vi "2D experiment kinect.vi"() -> ()   [LabVIEW 2011]
uses:
  <vilib>/Platform/TimedLoop/XDataNode/timing_clust.ctl
  <vilib>/Platform/TimedLoop/XDataNode/nitl_modes.ctl
  <vilib>/Platform/TimedLoop/XDataNode/wakeup.ctl
  <vilib>/Utility/cursorutil.llb/Set Cursor (Cursor ID).vi
  <vilib>/Utility/inputDevices.llb/closeMouse.vi
  <vilib>/Utility/inputDevices.llb/mouseAcquire.vi
  <vilib>/Utility/file.llb/Write To Spreadsheet File (DBL).vi
  <vilib>/Utility/file.llb/Write To Spreadsheet File (I64).vi
  <vilib>/Platform/TimedLoop/XDataNode/XDataNode.xnode
  User32.dll
  <vilib>/Platform/TimedLoop/XDataNode/XDNodeRunTimeDep.lvlib
  3D_Experiment/kinect-1-4/Kinect_API.lvlib
panel:
  in  "Far object filter 2":i32(slide)=26869 scale=0.0..4305.0
  out "click 2":bool
  in  "Replace with?":i32=60000
  out "stop":bool
  out "initial time":u32
  out "XY Graph":cluster{"Y":dbl[], "Y":dbl[]}[](graph)
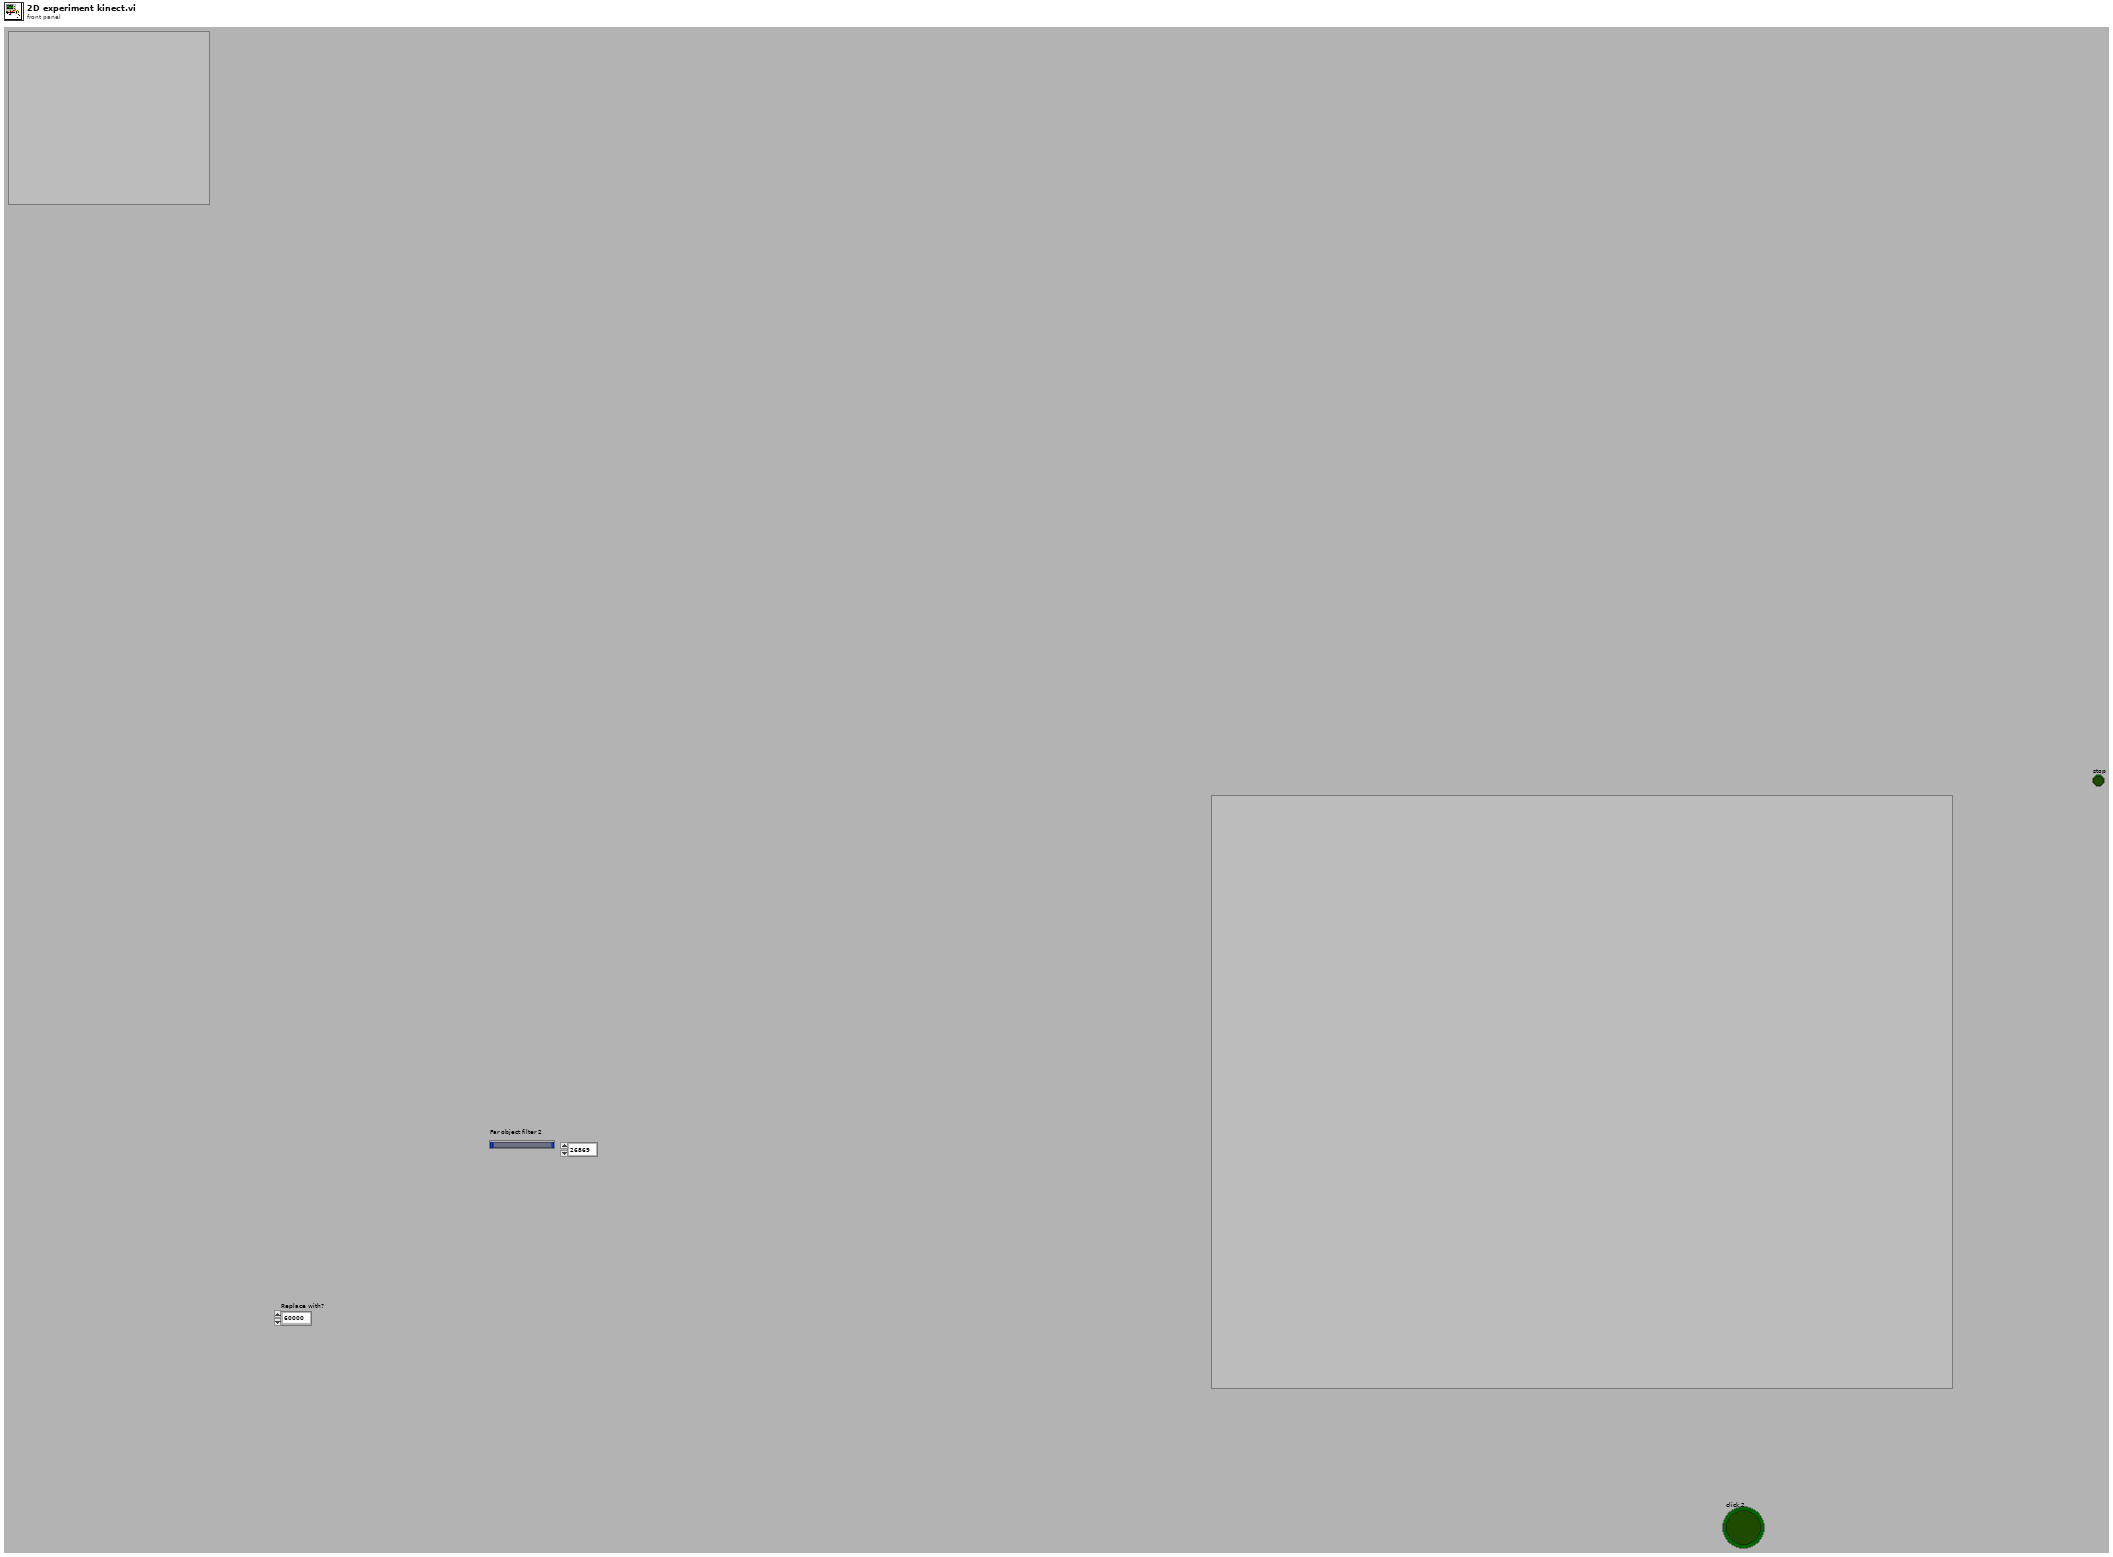
[diagram p1: front panel]
types:
  T1 = enum16{"open", "replace", "create", "open or create", "replace or create", "replace or create with confirmation"}
  T2 = typedef "XDNodeRunTimeDep.lvlib/timing_clust.ctl" = cluster{"Expected End [f-1]":u64, "Actual End [f-1]":u64, "Finished Late? [f-1]":bool, "Expected End [i-1]":u64, "Actual End [i-1]":u64, "Finished Late? [i-1]":bool, "Expected Start [i]":u64, "Actual Start [i]":u64, "Expected Start [f]":u64, "Actual Start [f]":u64, "Source Name":string, "Structure Name":string, "Period":i64, "Deadline":i64, "Offset":i64, "Start":i64, "Priority":i32, "Timeout":i32, "Mode":T3, "Wakeup Reason":T4, "Error":errorcluster, "Source Type":string, "Secondary Source Type":string, "Global End Time":u64, "Global Start Time":u64, "Frame Duration":u64, "Iteration Duration":u64, "Assigned CPU":i32, "I/O Scan Engine Mode":u32}
  T3 = typedef "XDNodeRunTimeDep.lvlib/nitl_modes.ctl" = enum32{"No Change", "Process missed periods, maintain original phase", "Discard missed periods, maintain original phase", "Process missed periods, ignore original phase", "Discard missed periods, ignore original phase"}
  T4 = typedef "XDNodeRunTimeDep.lvlib/wakeup.ctl" = enum32{"Normal", "Aborted", "Asynchronous wakeup", "Timing source error", "Timed loop error", "Timeout"}
  T5 = typedef "LVAllMonitorsDisplayTypeDef.ctl" = cluster{"Bounds":cluster{"Left":i16, "Top":i16, "Right":i16, "Bottom":i16}, "Depth":i16}[]
  T6 = cluster{"Bounds":cluster{"Left":i16, "Top":i16, "Right":i16, "Bottom":i16}, "Depth":i16}
  T7 = cluster{"Left":i16, "Top":i16, "Right":i16, "Bottom":i16}
  T8 = cluster{"queue out":refnum<queue>, "queue out":refnum<queue>}
  T9 = cluster{"new reference":refnum<k24>, "DepthStream":refnum<k24>, "VideoStream":refnum<k24>, "Event Callback":refnum<k27>, "Event Callback":refnum<k27>}
  T10 = cluster{"Horizontal":i32, "Vertical":i32, "Scrolling":i32}
  T11 = cluster{"button 1":bool, "button 2":bool, "button 3":bool, "button 4":bool}
  T12 = cluster{"Radius":dbl, "x0":dbl, "y0":dbl, "D":dbl, bool}
  T13 = typedef "LVPoint32TypeDef.ctl" = cluster{"Horizontal":i32, "Vertical":i32}
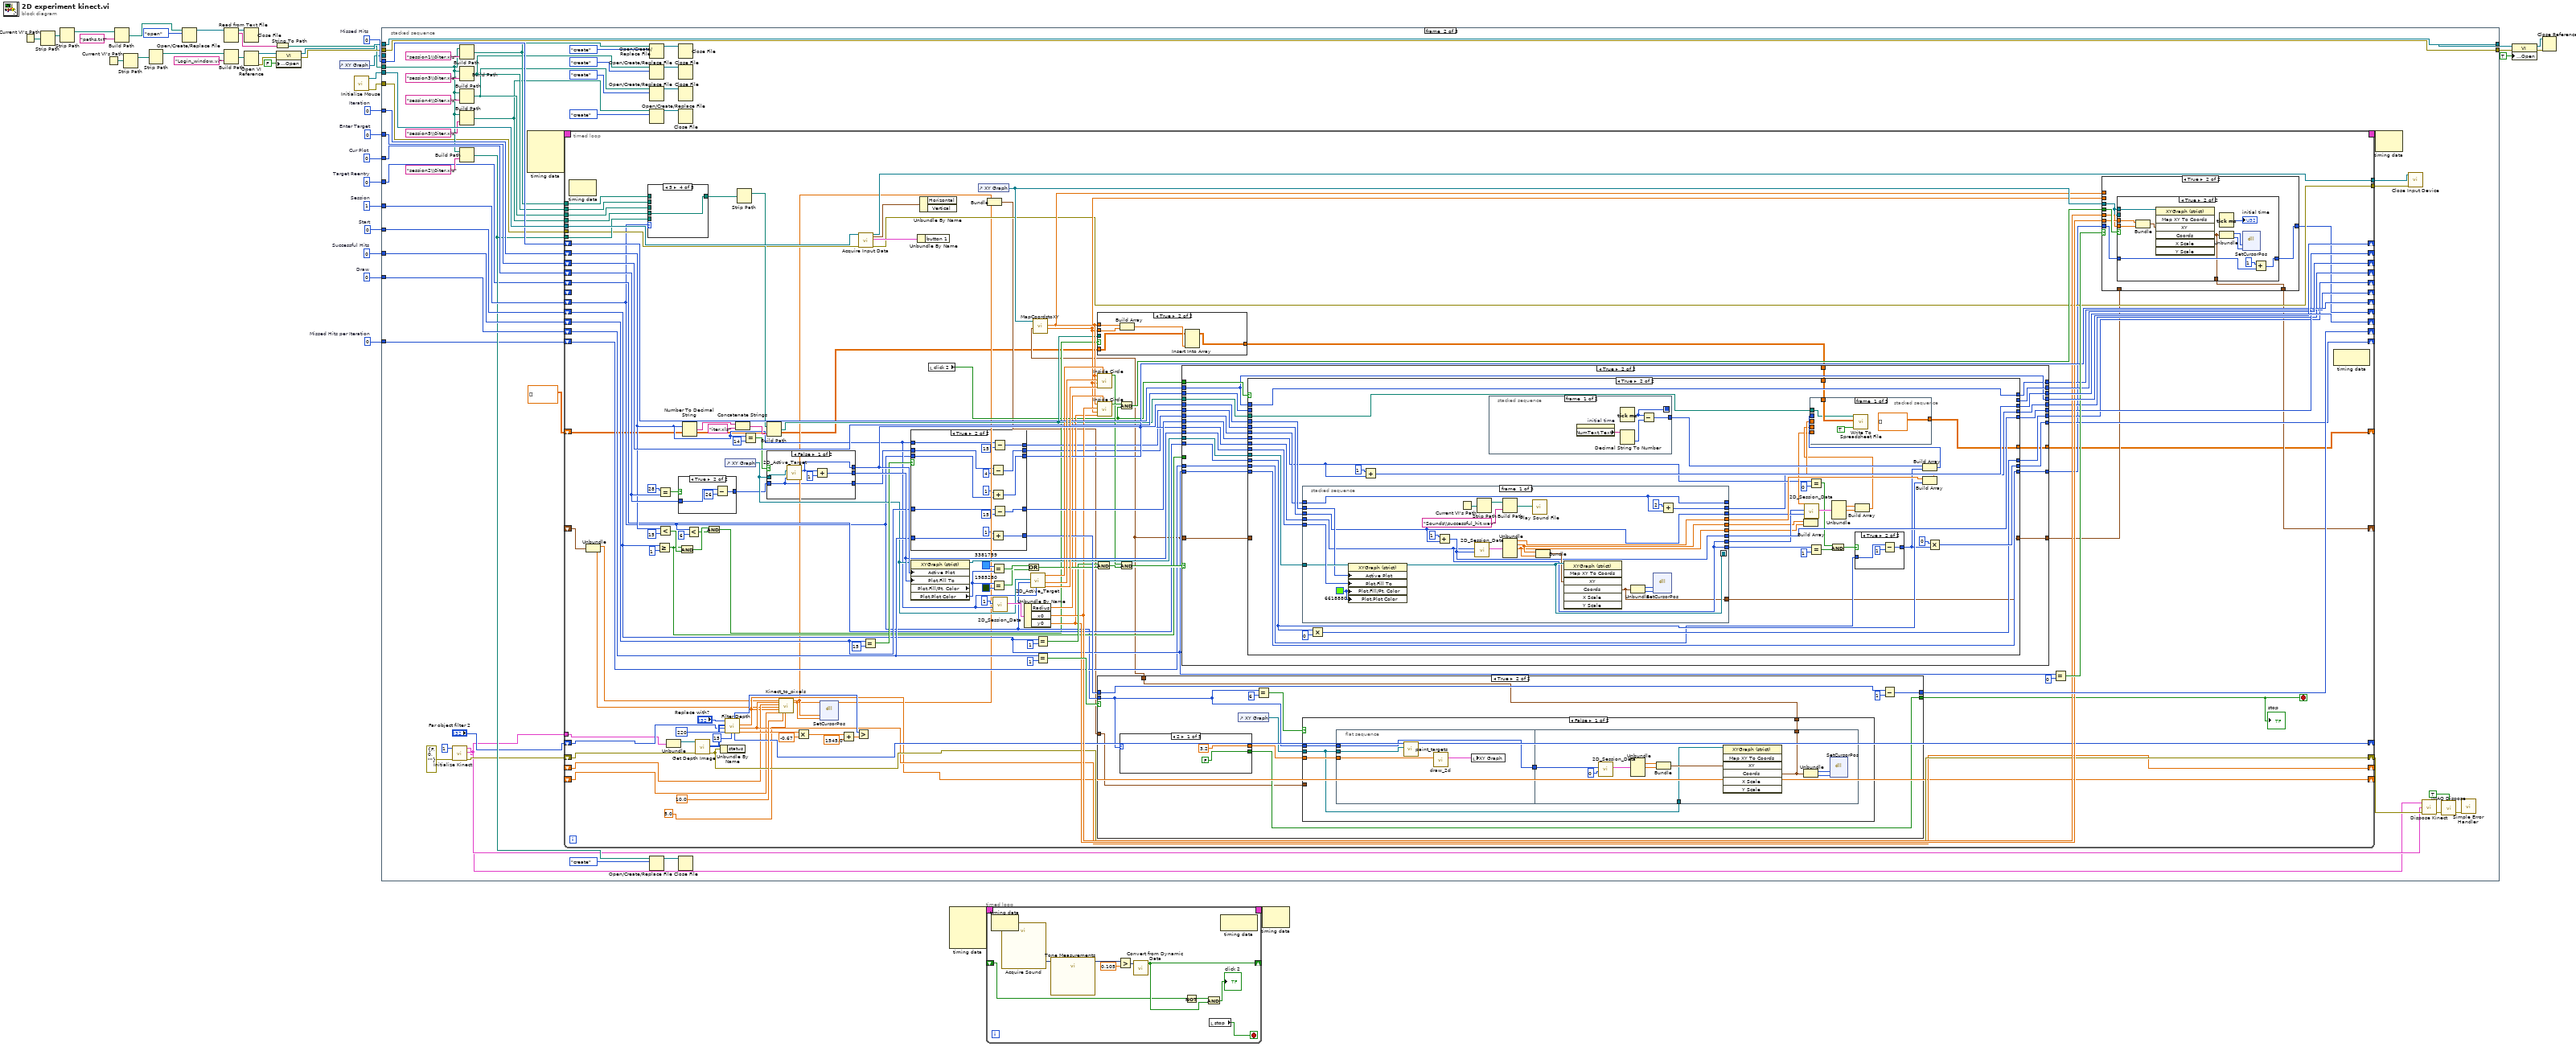
[diagram p0: block diagram]
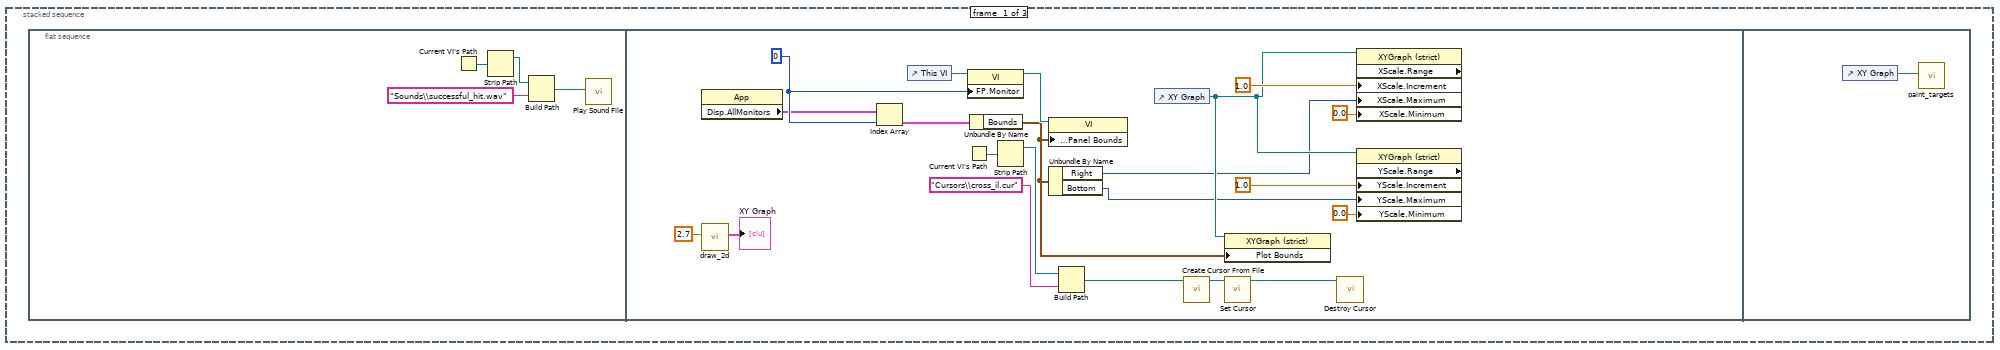
[diagram p2: hidden frame]
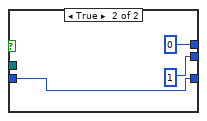
[diagram p8: hidden frame]
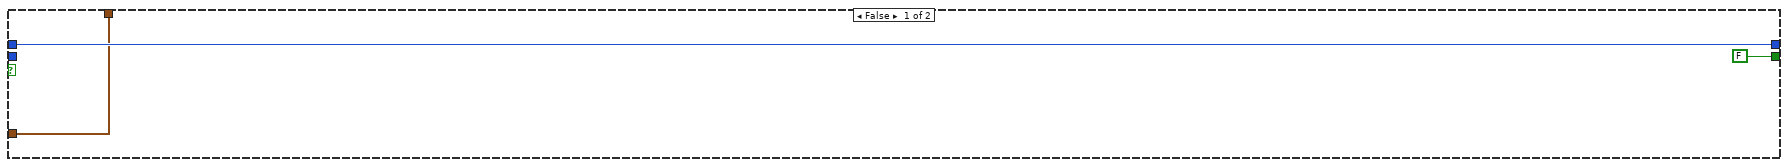
[diagram p10: hidden frame]
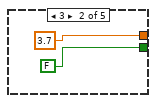
[diagram p12: hidden frame]
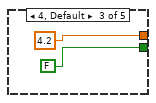
[diagram p13: hidden frame]
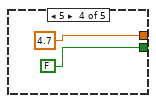
[diagram p14: hidden frame]
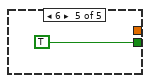
[diagram p15: hidden frame]
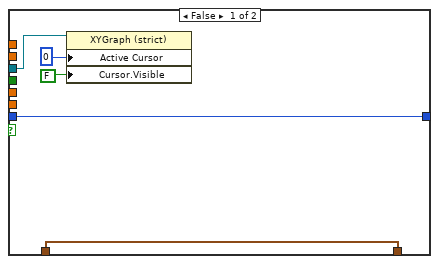
[diagram p16: hidden frame]
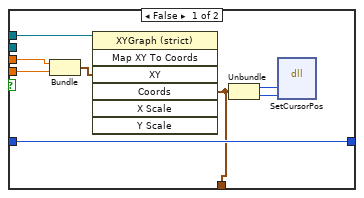
[diagram p17: hidden frame]
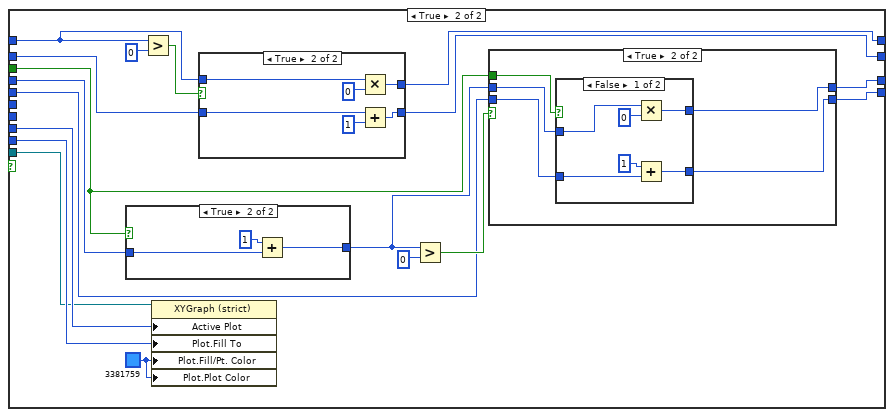
[diagram p20: hidden frame]
diagram:
  w3 = 0  # Target Reentry
  w4 = 0  # Missed Hits per Iteration
  w32 = 0  # Iteration
  w33 = 0  # Cur Plot
  w35 = 0  # Start
  w36 = 0  # Draw
  w37 = 1  # Session
  w38 = 0  # Successful Hits
  w39 = 0  # Missed Hits
  w40 = 0  # Enter Target
  n1 = Current VI's Path() -> (path=w13:path)
  n2 = Strip Path(path=w13) -> (stripped path=w8:path)  [unwired: 1 out]
  n3 = Strip Path(path=w8) -> (stripped path=w7:path)  [unwired: 1 out]
  n4 = Current VI's Path() -> (path=w28:path)
  n5 = Build Path(base path=w7, name or relative path="paths.txt") -> (appended path=w12:path)
  n6 = Strip Path(path=w28) -> (stripped path=w23:path)  [unwired: 1 out]
  n7 = Strip Path(path=w23) -> (stripped path=w22:path)  [unwired: 1 out]
  n8 = Open/Create/Replace File(file path (use dialog)=w12, operation (0:open)=T1."open") -> (refnum out=w15:refnum<file>)  [unwired: 4 in, 2 out]
  n9 = Read from Text File(file (use dialog)=w15) -> (refnum out=w16:refnum<file>, text=w14:string)  [unwired: 3 in, 2 out]
  n10 = Build Path(base path=w22, name or relative path="Login_window.vi") -> (appended path=w26:path)
  n11 = Close File(refnum=w16) -> ()  [unwired: 1 in, 2 out]
  n12 = Open VI Reference(vi path=w26) -> (vi reference=w31:refnum<vi>, error out=w30:errorcluster)  [unwired: 5 in]
  n13 = String To Path(string=w14) -> (path=w9:path)
  n14 = property class="VI"(reference=w31, error in=w30, "Front Panel Window:Open"=FALSE) -> (reference out=w25:refnum<vi>, error out=w24:errorcluster)
  n15 = control-ref of="XY Graph"() -> (w6:refnum<vi>)
  n16 = call <vilib>:"Initialize Mouse.vi"() -> ("error out"=w5:errorcluster, "device ID"=w34:refnum<k1>)  [unwired: 10 in]
  n17 = stacked-sequence {
    tunnel: w34 -> [_ w116 _]
    tunnel: w38 -> [_ w115 _]
    tunnel: w39 -> [_ w114 _]
    tunnel: w37 -> [_ w110 _]
    tunnel: w35 -> [_ w113 _]
    tunnel: w36 -> [_ w112 _]
    tunnel: w40 -> [_ w111 _]
    tunnel: w33 -> [_ w109 _]
    tunnel: w32 -> [_ w108 _]
    tunnel: w25 -> [_ w105 _]
    tunnel: w24 -> [_ w104 _]
    tunnel: [_ w105 _] -> w18
    tunnel: [_ w104 _] -> w17
    tunnel: w9 -> [_ w85 _]
    tunnel: w6 -> [_ _ w588]
    tunnel: w5 -> [_ w78 _]
    tunnel: w4 -> [_ w89 _]
    tunnel: w3 -> [_ w88 _]
    frame #0 {
      n18 = flat-sequence {
        frame #0 {
          n19 = Current VI's Path() -> (path=w42:path)
          n20 = Strip Path(path=w42) -> (stripped path=w43:path)  [unwired: 1 out]
          n21 = Build Path(base path=w43, name or relative path="Sounds\\successful_hit.wav") -> (appended path=w41:path)
          n22 = call <vilib>:"Play Sound File.vi"("path"=w41) -> ()  [unwired: 9 in, 2 out]
        }
        frame #1 {
          w61 = u16 0 ("Front Panel Window:Monitor")
          n23 = property class="App"() -> ("Disp.AllMonitors"=w60:T5)  [unwired: 2 in, 2 out]
          n24 = call "draw_2d.vi"("ID"=2.7) -> ("appended array"=→"XY Graph":cluster{dbl[], dbl[]}[])  [unwired: 10 in]
          n25 = Index Array(array=w60, index=w61) -> (element=w62:T6)
          n26 = control-ref of="This VI"() -> (w63:refnum<vi>)
          n27 = Current VI's Path() -> (path=w52:path)
          n28 = property class="VI"(reference=w63, "FP.Monitor"=w61) -> (reference out=w59:refnum<vi>)  [unwired: 1 in, 1 out]
          n29 = Unbundle By Name(w62) -> ("Bounds"=w58:T7)
          n30 = Strip Path(path=w52) -> (stripped path=w51:path)  [unwired: 1 out]
          n31 = property class="VI"(reference=w59, "Front Panel Window:Panel Bounds"=w58) -> ()  [unwired: 1 in, 2 out]
          n32 = Unbundle By Name(w58) -> ("Right"=w46:i16, "Bottom"=w45:i16)
          n33 = Build Path(base path=w51, name or relative path="Cursors\\cross_il.cur") -> (appended path=w49:path)
          n34 = control-ref of="XY Graph"() -> (w53:refnum<vi>)
          n35 = call <vilib>:"Create Cursor From File.vi"("cursor file"=w49) -> ("cursor ID"=w48:refnum<k1>)  [unwired: 9 in, 1 out]
          n36 = property on="Property Node" class="XYGraph (strict)"(reference=w53, "Plot Bounds"=w58) -> ()  [unwired: 1 in, 2 out]
          n37 = call-poly <vilib>:"Set Cursor.vi"("cursor ID"=w48) -> ("previous cursor ID"=w47:refnum<k1>)  [unwired: 9 in, 1 out]
          n38 = call <vilib>:"Destroy Cursor.vi"("cursor ID"=w47) -> ()  [unwired: 9 in, 1 out]
          n39 = property on="Property Node" class="XYGraph (strict)" props=["XScale", "Range", "XScale", "Increment", "XScale", "Maximum", "XScale", "Minimum"](reference=w53, "XScale.Increment"=1.0 ("X Scale.Range:Increment"), "XScale.Maximum"=w46, "XScale.Minimum"=0.0 ("X Scale.Range:Minimum")) -> ()  [unwired: 1 in, 3 out]
          n40 = property on="Property Node" class="XYGraph (strict)" props=["YScale", "Range", "YScale", "Increment", "YScale", "Maximum", "YScale", "Minimum"](reference=w53, "YScale.Increment"=1.0 ("Y Scale.Range:Increment"), "YScale.Maximum"=w45, "YScale.Minimum"=0.0 ("Y Scale.Range:Minimum")) -> ()  [unwired: 1 in, 3 out]
        }
        frame #2 {
          n41 = control-ref of="XY Graph"() -> (w66:refnum<vi>)
          n42 = call "paint_targets.vi"("XYGraph Refnum"=w66) -> ()  [unwired: 11 in]
        }
      }
    }
    frame #1 {
      n43 = call "Initialize Kinect.vi"("error in (no error)"=errorcluster {"status"=FALSE, "code"=0, "source"=""}, "Buffer Size"=1) -> ("error out"=w71:errorcluster, "Queues Out"=w69:T8, "References"=w68:T9)  [unwired: 7 in]
      n44 = Build Path(base path=w85, name or relative path="session1\\0iter.xls") -> (appended path=w98:path)
      n45 = Build Path(base path=w85, name or relative path="session3\\0iter.xls") -> (appended path=w92:path)
      n46 = Build Path(base path=w85, name or relative path="session4\\0iter.xls") -> (appended path=w82:path)
      n47 = Build Path(base path=w85, name or relative path="session5\\0iter.xls") -> (appended path=w79:path)
      n48 = Build Path(base path=w85, name or relative path="session2\\0iter.xls") -> (appended path=w95:path)
      n49 = node-c288() -> (w107:T2)  [unwired: 4 in]
      n50 = timed-loop {
        tunnel: w116 -> [w233]
        tunnel: [w232] -> w91
        shift-right: [w231] -> _
        shift-left: w115 -> [w218]
        shift-right: [w229] -> _
        shift-left: w114 -> [w230]
        shift-right: [w210] -> _
        shift-left: w110 -> [w158]
        shift-right: [w160] -> _
        shift-left: w113 -> [w179]
        shift-right: [w215] -> _
        shift-left: w112 -> [w216]
        shift-right: [w211] -> _
        shift-left: w111 -> [w212]
        shift-right: [w196] -> _
        shift-left: w108 -> [w170]
        shift-right: [w195] -> _
        shift-left: w109 -> [w192]
        timing: w107 -> [_]
        timing-out: [_] -> w106
        tunnel: w98 -> [w185]
        tunnel: w95 -> [w184]
        tunnel: w92 -> [w183]
        shift-right: [w172] -> _
        shift-left: _ -> [_]
        tunnel: w78 -> [w168]
        tunnel: [w167] -> w90
        shift-right: [w165] -> _
        shift-left: w89 -> [w166]
        shift-right: [w162] -> _
        shift-left: w88 -> [w164]
        tunnel: w82 -> [w154]
        tunnel: w79 -> [w153]
        shift-right: [w138] -> w72
        shift-left: w71 -> [w137]
        shift-right: [w136] -> _
        shift-left: "Far object filter 2" -> [w135]
        tunnel: w69 -> [w134]
        shift-right: [w133] -> _
        shift-left: _ -> [w132]
        shift-right: [w131] -> _
        shift-left: _ -> [w130]
        shift-right: [w124] -> _
        shift-left: _ -> [w123]
        shift-right: [w117] -> _
        shift-left: dbl[][] [] -> [w119]
        stop <- w152 stop-if-true
        n51 = node-c288() -> ()  [unwired: 1 in, 1 out]
        n52 = Unbundle(w123) -> ("X_pixels"=w122:dbl, "Y_pixels"=w121:dbl)
        n53 = case shown="5" w158 {
          tunnel: w185 -> [_ _ _ _ w254]
          tunnel: [w250 w251 w252 w253 w254] -> w178
          tunnel: w184 -> [w250 _ _ _ _]
          tunnel: w183 -> [_ w251 _ _ _]
          tunnel: w154 -> [_ _ w252 _ _]
          tunnel: w153 -> [_ _ _ w253 _]
          frame 2 {
          }
          frame 3 {
          }
          frame 4 {
          }
          frame 5 {
          }
          frame 1, Default {
          }
        }
        n54 = Greater Or Equal?(x=w179, y=1) -> (x >= y?=w163:bool)
        n55 = Equal?(x=28, y=w192) -> (x = y?=w193:bool)
        n56 = Less?(x=w170, y=15) -> (x < y?=w169:bool)
        n57 = Unbundle(w134) -> ("queue out"=w139:refnum<queue>)  [unwired: 1 out]
        n58 = case shown="True" w193 {
          tunnel: w192 -> [w265 w268]
          tunnel: [w265 w266] -> w191
          frame False {
          }
          frame True {
            n59 = Subtract(x=w268, y=26) -> (x-y=w266:i32)
          }
        }
        n60 = And(x=w163, y=w169) -> (x .and. y?=w159:bool)
        n61 = Number To Decimal String(number=w170) -> (decimal integer string=w174:string)  [unwired: 1 in]
        n62 = Less?(x=w158, y=6) -> (x < y?=w156:bool)
        n63 = call "Get Depth Image.vi"("error in (no error)"=w137, "queue in"=w139) -> ("error out"=w138:errorcluster, "Depth Image Pixels (U16)"=w141:u16[][])  [unwired: 6 in, 2 out]
        n64 = And(x=w159, y=w156) -> (x .and. y?=w155:bool)
        n65 = Unbundle By Name(w138) -> ()  [unwired: 1 out]
        n66 = control-ref of="XY Graph"() -> (w199:refnum<vi>)
        n67 = call "Filter Depth.vi"("Wall-Threshold"=15, "Y-Threshold"=220, "Far object filter"=w135, "Depth Image Pixels (U16)"=w141, "Replace with?"="Replace with?") -> ("average Z"=w147:dbl, "average Y"=w133:dbl, "average X"=w131:dbl, "New far object filter"=w136:i32, "Area"=w148:i32)  [unwired: 1 in, 1 out]
        n68 = Concatenate Strings(w174, "iter.xls" ("name or relative path")) -> (w176:string)
        n69 = Strip Path(path=w178) -> (stripped path=w175:path)  [unwired: 1 out]
        n70 = Equal?(x=w170, y=14) -> (x = y?=w189:bool)
        n71 = Build Path(base path=w175, name or relative path=w176) -> (appended path=w173:path)
        n72 = case shown="False" w189 {
          tunnel: [w260 u32 0 ("Active Plot")] -> w238
          tunnel: [w259 u32 1] -> w237
          tunnel: w199 -> [w258 _]
          tunnel: w191 -> [w257 w262]
          tunnel: [w257 w262] -> w188
          frame False {
            n73 = call "2D_Active_Target.vi"("Active Plot"=w257, "XYGraph Refnum"=w258) -> ("Active Plot"=w260:u32)  [unwired: 6 in, 3 out]
            n74 = Add(x=w260, y=u32 1) -> (x+y=w259:u32)
          }
          frame True {
          }
        }
        n75 = call "Kinect_to_pixels.vi"("previous_X_pixels"=w122, "current_X_kinect"=w133, "previous_X_kinect"=w132, "previous_Y_pixels"=w121, "current_Y_kinect"=w131, "previous_Y_kinect"=w130, "X_Y_speed"=10.0, "min_diff"=5.0) -> ("X_pixels"=w129:dbl, "Y_pixels"=w128:dbl)  [unwired: 8 in, 2 out]
        n76 = Multiply(x=w147, y=-0.67 ("x")) -> (x*y=w143:dbl)
        n77 = dll-call lib="User32.dll" fn="SetCursorPos"(w129, w128) -> ()  [unwired: 6 in, 2 out]
        n78 = Add(x=w143, y=1545.0 ("x")) -> (x+y=w144:dbl)
        n79 = Greater?(x=w148, y=w144) -> ()  [unwired: 1 out]
        n80 = call-poly <vilib>:"Acquire Input Data.vi"("device ID"=w233, "error in (no error)"=w168) -> ("device ID"=w232:refnum<k1>, "axis info"=w198:T10, "button info"=w234:T11, "error out"=w167:errorcluster)  [unwired: 1 in, 13 out]
        n81 = Equal?(x=w218, y=15) -> (x = y?=w227:bool)
        n82 = case shown="True" w227 {
          tunnel: w218 -> [w347 w362]
          tunnel: [w347 w361] -> w226
          tunnel: w158 -> [w346 w360]
          tunnel: [w346 w358] -> w210
          tunnel: w216 -> [w345 w357]
          tunnel: [w345 w355] -> w214
          tunnel: w188 -> [w344 w354]
          tunnel: [w344 w352] -> w187
          tunnel: w170 -> [w343 w351]
          tunnel: [w343 w349] -> w186
          frame False {
          }
          frame True {
            n83 = Subtract(x=w354, y=4) -> (x-y=w352:i32)
            n84 = Add(x=1, y=w360) -> (x+y=w358:i32)
            n85 = Add(x=1, y=w357) -> (x+y=w355:i32)
            n86 = Subtract(x=w351, y=15) -> (x-y=w349:i32)
            n87 = Subtract(x=w362, y=15) -> (x-y=w361:i32)
          }
        }
        n88 = property on="Property Node" class="XYGraph (strict)" props=["Active Plot", "Plot", "Fill To", "Plot", "Fill/Pt. Color", "Plot", "Plot Color"](reference=w199, "Active Plot"=w238, "Plot.Fill To"=w237) -> (reference out=w219:refnum<vi>, "Plot.Plot Color"=w220:u32)  [unwired: 1 in, 2 out]
        n89 = Unbundle By Name(w234) -> ()  [unwired: 1 out]
        n90 = Unbundle By Name(w198) -> ()  [unwired: 2 out]
        n91 = local read "click 2"() -> (w151:bool)
        n92 = control-ref of="XY Graph"() -> (w197:refnum<vi>)
        n93 = Bundle("X_pixels"=w129, "Y_pixels"=w128) -> (w127:cluster{"X_pixels":dbl, "Y_pixels":dbl})  [unwired: 1 in]
        n94 = Equal?(x=u32 3381759, y=w220) -> (x = y?=w240:bool)
        n95 = Equal?(x=w220, y=u32 1985280) -> (x = y?=w239:bool)
        n96 = call "2D_Session_Data.vi"("Iteration"=w170, "Session"=1) -> ("output cluster"=w204:T12)  [unwired: 9 in]
        n97 = Unbundle By Name(w204) -> ("Radius"=w203:dbl, "x0"=w202:dbl, "y0"=w201:dbl)
        n98 = Or(x=w240, y=w239) -> (x .or. y?=w208:bool)
        n99 = call "2D_Active_Target.vi"("Iteration"=w170, "Session"=w158, "XYGraph Refnum"=w199) -> ("y0"=w235:dbl, "x0"=w236:dbl, "Radius"=w225:dbl)  [unwired: 5 in, 1 out]
        n100 = Equal?(x=w179, y=1) -> (x = y?=w206:bool)
        n101 = Equal?(x=w216, y=1) -> (x = y?=w213:bool)
        n102 = And(x=w206, y=w208) -> (x .and. y?=w205:bool)
        n103 = case shown="True" w213 {
          tunnel: w158 -> [_ w274]
          tunnel: [w270 w281] -> w215
          tunnel: w214 -> [w270 w280]
          tunnel: [FALSE ("Valid") w278] -> w152
          tunnel: w127 -> [w269 w272]
          tunnel: [w269 w273] -> w126
          frame False {
          }
          frame True {
            n104 = case shown="2" w274 {
              tunnel: [3.2 ("ID") 3.7 ("ID") 4.2 ("ID") 4.7 ("ID") _] -> w279
              tunnel: [FALSE FALSE FALSE FALSE TRUE] -> w278
              frame 2 {
              }
              frame 3 {
              }
              frame 4, Default {
              }
              frame 5 {
              }
              frame 6 {
              }
            }
            n105 = control-ref of="XY Graph"() -> (w275:refnum<vi>)
            n106 = Equal?(x=w274, y=6) -> (x = y?=w276:bool)
            n107 = case shown="False" w276 {
              tunnel: w279 -> [w287 _]
              tunnel: w275 -> [w284 _]
              tunnel: w274 -> [w285 _]
              tunnel: [w283 w302] -> w273
              tunnel: w272 -> [_ w302]
              frame False {
                n108 = flat-sequence {
                  tunnel: w287 -> [w290]
                  tunnel: w284 -> [w289]
                  tunnel: [w288] -> w286
                  tunnel: w285 -> [w288]
                  tunnel: w286 -> [w295]
                  tunnel: w284 -> [w293]
                  tunnel: [w292] -> w283
                  frame #0 {
                    n109 = call "paint_targets.vi"("XYGraph Refnum"=w289) -> ()  [unwired: 11 in]
                    n110 = call "draw_2d.vi"("ID"=w290) -> ("appended array"=w291:cluster{dbl[], dbl[]}[])  [unwired: 10 in]
                    n111 = local write "XY Graph"(w291) -> ()
                  }
                  frame #1 {
                    n112 = call "2D_Session_Data.vi"("Iteration"=0, "Session"=w295) -> ("output cluster"=w299:T12)  [unwired: 9 in]
                    n113 = Unbundle(w299) -> ("x0"=w298:dbl, "y0"=w296:dbl)  [unwired: 3 out]
                    n114 = Bundle("x0"=w298, "y0"=w296) -> (w297:cluster{"x0":dbl, "y0":dbl})  [unwired: 1 in]
                    n115 = invoke on="Invoke Node" class="XYGraph (strict)" method="Map XY To Coords"(reference=w293, "XY"=w297) -> ("Coords"=w292:T13)  [unwired: 5 in, 6 out]
                    n116 = Unbundle(w292) -> ("Horizontal"=w301:i32, "Vertical"=w300:i32)
                    n117 = dll-call lib="User32.dll" fn="SetCursorPos"(w301, w300) -> ()  [unwired: 6 in, 2 out]
                  }
                }
              }
              frame True {
              }
            }
            n118 = Subtract(x=w280, y=1) -> (x-y=w281:i32)
          }
        }
        "stop" <- w152
        n119 = call "MapCoordstoXY.vi"("Coordinates"=w126, "XYGraph Refnum"=w197) -> ("Y(graph)"=w181:dbl, "X (graph)"=w182:dbl)  [unwired: 7 in]
        n120 = case shown="True" w155 {
          tunnel: w182 -> [_ w249]
          tunnel: w181 -> [_ w248]
          tunnel: w173 -> [_ _]
          tunnel: w119 -> [w244 w246]
          tunnel: [w244 w245] -> w118
          frame False {
          }
          frame True {
            n121 = Build Array(w249, w248) -> (w247:dbl[])
            n122 = Insert Into Array(array=w246, new element=w247) -> (w245:dbl[][])  [unwired: 2 in]
          }
        }
        n123 = call "Inside Circle.vi"("Radius"=w225, "y0"=w235, "y"=w181, "x0"=w236, "x"=w182) -> ("Inside Circle"=w207:bool)  [unwired: 6 in]
        n124 = call "Inside Circle.vi"("Radius"=w203, "y0"=w201, "y"=w181, "x0"=w202, "x"=w182) -> ("Inside Circle"=w222:bool)  [unwired: 6 in]
        n125 = And(x=w222, y=w151) -> (x .and. y?=w221:bool)
        n126 = And(x=w207, y=w205) -> (x .and. y?=w242:bool)
        n127 = case shown="True" w242 {
          tunnel: w151 -> [w373 w456]
          tunnel: w238 -> [w381 w453]
          tunnel: w237 -> [w380 w452]
          tunnel: w226 -> [w365 w455]
          tunnel: [w365 w454] -> w231
          tunnel: w230 -> [w375 w440]
          tunnel: [w371 w440] -> w229
          tunnel: w179 -> [w379 w451]
          tunnel: [w379 w450] -> w161
          tunnel: w219 -> [w378 w449]
          tunnel: w212 -> [w370 w448]
          tunnel: [_ w447] -> w211
          tunnel: w210 -> [w366 w446]
          tunnel: w186 -> [w377 w445]
          tunnel: [w377 w444] -> w196
          tunnel: w187 -> [w376 w443]
          tunnel: [w376 w442] -> w195
          tunnel: w173 -> [_ w441]
          tunnel: [w375 w439] -> w172
          tunnel: w166 -> [w374 w438]
          tunnel: [w372 w437] -> w165
          tunnel: w164 -> [w368 w436]
          tunnel: w163 -> [w369 _]
          tunnel: [w367 w435] -> w162
          tunnel: w126 -> [w364 w434]
          tunnel: [w364 w433] -> w125
          tunnel: w118 -> [w363 w432]
          tunnel: [w363 w431] -> w117
          frame False {
            n128 = case shown="False" w369 {
              tunnel: w381 -> [_ w402]
              tunnel: w380 -> [_ w401]
              tunnel: w378 -> [_ w400]
              tunnel: w375 -> [w385 w399]
              tunnel: w374 -> [w384 w395]
              tunnel: w373 -> [_ w386]
              tunnel: [w384 w394] -> w372
              tunnel: [w385 w393] -> w371
              tunnel: w370 -> [w382 w390]
              tunnel: w368 -> [w383 w389]
              tunnel: [w383 w388] -> w367
              tunnel: [w382 w387] -> _
              tunnel: w366 -> [_ _]
              tunnel: w365 -> [_ _]
              frame False {
              }
              frame True {
                w403 = u32 3381759
                n129 = case shown="True" w386 {
                  tunnel: w399 -> [w427 w430]
                  tunnel: [w427 w428] -> w396
                  frame False {
                  }
                  frame True {
                    n130 = Add(x=1, y=w430) -> (x+y=w428:i32)
                  }
                }
                n131 = Greater?(x=w390, y=0) -> (0:w391:bool)
                n132 = property on="Property Node" class="XYGraph (strict)"(reference=w400, "Active Plot"=w402, "Plot.Fill To"=w401, "Plot.Fill/Pt. Color"=w403, "Plot.Plot Color"=w403) -> ()  [unwired: 1 in, 2 out]
                n133 = case shown="True" w391 {
                  tunnel: w390 -> [w404 w411]
                  tunnel: w389 -> [w405 w408]
                  tunnel: [w405 w407] -> w388
                  tunnel: [w404 w406] -> w387
                  frame False {
                  }
                  frame True {
                    n134 = Multiply(x=w411, y=0) -> (x*y=w406:i32)
                    n135 = Add(x=w408, y=1) -> (x+y=w407:i32)
                  }
                }
                n136 = Greater?(x=w396, y=0) -> (0:w397:bool)
                n137 = case shown="True" w397 {
                  tunnel: [w412 w418] -> w394
                  tunnel: [w413 w417] -> w393
                  tunnel: w396 -> [w413 w416]
                  tunnel: w395 -> [w412 w415]
                  tunnel: w386 -> [_ w414]
                  frame False {
                  }
                  frame True {
                    n138 = case shown="False" w414 {
                      tunnel: [w423 w425] -> w418
                      tunnel: [w421 w426] -> w417
                      tunnel: w416 -> [w420 w426]
                      tunnel: w415 -> [w419 w425]
                      frame False {
                        n139 = Multiply(x=w420, y=0) -> (x*y=w421:i32)
                        n140 = Add(x=1, y=w419) -> (x+y=w423:i32)
                      }
                      frame True {
                      }
                    }
                  }
                }
              }
            }
          }
          frame True {
            n141 = case shown="True" w456 {
              tunnel: w455 -> [w471 w485]
              tunnel: [w471 w510] -> w454
              tunnel: w453 -> [w470 w514]
              tunnel: w452 -> [w469 w513]
              tunnel: w451 -> [w468 w512]
              tunnel: [w468 w512] -> w450
              tunnel: w449 -> [w467 w511]
              tunnel: w448 -> [w466 _]
              tunnel: [w464 _] -> w447
              tunnel: w446 -> [_ w509]
              tunnel: w445 -> [w463 w508]
              tunnel: [w463 w507] -> w444
              tunnel: w443 -> [w462 w506]
              tunnel: [w462 w476] -> w442
              tunnel: w441 -> [_ w503]
              tunnel: w440 -> [w461 w502]
              tunnel: [w461 w502] -> w439
              tunnel: w438 -> [w460 w478]
              tunnel: [w460 w501] -> w437
              tunnel: w436 -> [w459 w498]
              tunnel: [w459 w496] -> w435
              tunnel: w434 -> [w458 _]
              tunnel: [w458 w475] -> w433
              tunnel: w432 -> [w457 w474]
              tunnel: [w457 w473] -> w431
              frame False {
                w472 = u32 1985280
                n142 = property on="Property Node" class="XYGraph (strict)"(reference=w467, "Active Plot"=w470, "Plot.Fill To"=w469, "Plot.Fill/Pt. Color"=w472, "Plot.Plot Color"=w472) -> ()  [unwired: 1 in, 2 out]
                n143 = Add(x=w466, y=1) -> (x+y=w464:i32)
              }
              frame True {
                n144 = stacked-sequence {
                  seq-local: [w562 _ _] -> [_ w571 w582]
                  tunnel: w514 -> [w561 w570 w584]
                  tunnel: w513 -> [w564 _ w583]
                  tunnel: w511 -> [w563 _ _]
                  tunnel: w509 -> [w543 _ _]
                  tunnel: w508 -> [w546 w569 _]
                  tunnel: [w548 _ _] -> w507
                  tunnel: [w555 _ _] -> _
                  tunnel: w506 -> [w555 _ _]
                  tunnel: [w553 _ _] -> w476
                  tunnel: [w547 _ _] -> w499
                  tunnel: [w546 _ _] -> w494
                  tunnel: [w543 _ _] -> w493
                  tunnel: [w545 _ _] -> w489
                  tunnel: [w544 _ _] -> w488
                  tunnel: [w543 _ _] -> w483
                  tunnel: [w542 _ _] -> w475
                  frame #0 {
                    w565 = u32 6618880
                    n145 = property on="Property Node" class="XYGraph (strict)"(reference=w563, "Active Plot"=w561, "Plot.Fill To"=w564, "Plot.Fill/Pt. Color"=w565, "Plot.Plot Color"=w565) -> (reference out=w562:refnum<vi>)  [unwired: 1 in, 1 out]
                    n146 = Add(x=1, y=w546) -> (x+y=w548:i32)
                    n147 = Current VI's Path() -> (path=w558:path)
                    n148 = call "2D_Session_Data.vi"("Iteration"=w548, "Session"=w543) -> ("output cluster"=w550:T12)  [unwired: 9 in]
                    n149 = Strip Path(path=w558) -> (stripped path=w557:path)  [unwired: 1 out]
                    n150 = Build Path(base path=w557, name or relative path="Sounds\\successful_hit.wav") -> (appended path=w559:path)
                    n151 = Unbundle(w550) -> ("Radius"=w547:dbl, "x0"=w545:dbl, "y0"=w544:dbl)  [unwired: 2 out]
                    n152 = call <vilib>:"Play Sound File.vi"("path"=w559) -> ()  [unwired: 9 in, 2 out]
                    n153 = Bundle("x0"=w545, "y0"=w544) -> (w549:cluster{"x0":dbl, "y0":dbl})  [unwired: 1 in]
                    n154 = invoke on="Invoke Node" class="XYGraph (strict)" method="Map XY To Coords"(reference=w562, "XY"=w549) -> ("Coords"=w542:T13)  [unwired: 5 in, 6 out]
                    n155 = Unbundle(w542) -> ("Horizontal"=w552:i32, "Vertical"=w551:i32)
                    n156 = dll-call lib="User32.dll" fn="SetCursorPos"(w552, w551) -> ()  [unwired: 6 in, 2 out]
                    n157 = Add(x=2, y=w555) -> (x+y=w553:i32)
                  }
                  frame #1 {
                    w573 = u32 3381759
                    n158 = Equal?(x=15, y=w569) -> (x = y?=w567:bool)
                    n159 = case shown="True" w567 {
                      tunnel: [w575 w579] -> w572
                      tunnel: w570 -> [w574 w581]
                      tunnel: [w574 w577] -> w566
                      frame False {
                        n160 = Add(x=w574, y=u32 1) -> (x+y=w575:u32)
                      }
                      frame True {
                        n161 = Subtract(x=w581, y=u32 2) -> (x-y=w577:u32)
                        n162 = Add(x=w577, y=1 ("x")) -> (x+y=w579:u32)
                      }
                    }
                    n163 = property on="Property Node" class="XYGraph (strict)"(reference=w571, "Active Plot"=w566, "Plot.Fill To"=w572, "Plot.Fill/Pt. Color"=w573, "Plot.Plot Color"=w573) -> ()  [unwired: 1 in, 2 out]
                  }
                  frame #2 {
                    w585 = u32 3223857
                    n164 = property on="Property Node" class="XYGraph (strict)"(reference=w582, "Active Plot"=w584, "Plot.Fill To"=w583, "Plot.Fill/Pt. Color"=w585, "Plot.Plot Color"=w585) -> ()  [unwired: 1 in, 2 out]
                  }
                }
                n165 = Multiply(x=w498, y=0) -> (x*y=w496:i32)
                n166 = Add(x=1, y=w485) -> (x+y=w510:i32)
                n167 = stacked-sequence {
                  seq-local: [w536 _] -> [_ w540]
                  tunnel: [w537 _] -> w504
                  frame #0 {
                    n168 = property on="initial time" class="DigNum (strict)"() -> ("NumText.Text"=w539:string)  [unwired: 2 in, 2 out]
                    n169 = Tick Count (ms)() -> (millisecond timer value=w536:u32)
                    n170 = Decimal String To Number(string=w539) -> (number=w538:i32)  [unwired: 2 in, 1 out]
                    n171 = Subtract(x=w536, y=w538) -> (x-y=w537:u32)
                  }
                  frame #1 {
                    n172 = Number To Decimal String(number=w540) -> (decimal integer string=w541:string)  [unwired: 1 in]
                    n173 = property on="initial time" class="DigNum (strict)"("NumText.Text"=w541) -> ()  [unwired: 2 in, 2 out]
                  }
                }
                n174 = Build Array(w489, w488) -> (w486:dbl[])
                n175 = call "2D_Session_Data.vi"("Iteration"=w494, "Session"=w493) -> ("output cluster"=w492:T12)  [unwired: 9 in]
                n176 = Equal?(x=w485, y=0) -> (x = y?=w481:bool)
                n177 = Equal?(x=w483, y=1) -> (x = y?=w480:bool)
                n178 = And(x=w481, y=w480) -> (x .and. y?=w479:bool)
                n179 = Unbundle(w492) -> ("x0"=w491:dbl, "y0"=w490:dbl)  [unwired: 3 out]
                n180 = Build Array(w491, w490) -> (w487:dbl[])
                n181 = case shown="True" w479 {
                  tunnel: w478 -> [w516 w518]
                  tunnel: [w516 w517] -> w477
                  frame False {
                  }
                  frame True {
                    n182 = Subtract(x=w518, y=1) -> (x-y=w517:i32)
                  }
                }
                n183 = Build Array(w504, w477) -> (w505:u32[])
                n184 = Build Array(w499, w498) -> (w495:dbl[])
                n185 = stacked-sequence {
                  tunnel: w505 -> [_ w526 _ _ _]
                  tunnel: w503 -> [w521 w524 w527 w532 w534]
                  tunnel: w495 -> [_ _ w529 _ _]
                  tunnel: w487 -> [_ _ _ w531 _]
                  tunnel: w486 -> [_ _ _ _ w535]
                  tunnel: w474 -> [w522 _ _ _ _]
                  tunnel: [dbl[][] [] _ _ _ _] -> w473
                  frame #0 {
                    n186 = call-poly <vilib>:"Write To Spreadsheet File.vi"("append to file? (new file:F)"=TRUE, "2D data"=w522, "file path (dialog if empty)"=w521) -> ()  [unwired: 5 in, 1 out]
                  }
                  frame #1 {
                    n187 = call-poly <vilib>:"Write To Spreadsheet File.vi"("append to file? (new file:F)"=TRUE, "1D data"=w526, "file path (dialog if empty)"=w524) -> ()  [unwired: 5 in, 1 out]
                  }
                  frame #2 {
                    n188 = call-poly <vilib>:"Write To Spreadsheet File.vi"("append to file? (new file:F)"=TRUE, "1D data"=w529, "file path (dialog if empty)"=w527) -> ()  [unwired: 5 in, 1 out]
                  }
                  frame #3 {
                    n189 = call-poly <vilib>:"Write To Spreadsheet File.vi"("append to file? (new file:F)"=TRUE, "1D data"=w531, "file path (dialog if empty)"=w532) -> ()  [unwired: 5 in, 1 out]
                  }
                  frame #4 {
                    n190 = call-poly <vilib>:"Write To Spreadsheet File.vi"("append to file? (new file:F)"=TRUE, "1D data"=w535, "file path (dialog if empty)"=w534) -> ()  [unwired: 5 in, 1 out]
                  }
                }
                n191 = Multiply(x=0, y=w477) -> (x*y=w501:i32)
              }
            }
          }
        }
        n192 = Equal?(x=w179, y=0) -> (x = y?=w223:bool)
        n193 = case shown="True" w223 {
          tunnel: w197 -> [w313 w318]
          tunnel: w182 -> [_ _]
          tunnel: w181 -> [_ _]
          tunnel: w221 -> [_ w323]
          tunnel: w161 -> [w316 w322]
          tunnel: [w316 w321] -> w160
          tunnel: w202 -> [_ w320]
          tunnel: w201 -> [_ w319]
          tunnel: w125 -> [w312 _]
          tunnel: [w312 w317] -> w124
          frame False {
            n194 = property on="Property Node" class="XYGraph (strict)"(reference=w313, "Active Cursor"=u32 0, "Cursor.Visible"=FALSE) -> ()  [unwired: 1 in, 2 out]
          }
          frame True {
            n195 = case shown="True" w323 {
              tunnel: w322 -> [w331 w338]
              tunnel: [w331 w337] -> w321
              tunnel: w320 -> [w327 w342]
              tunnel: w319 -> [w326 w341]
              tunnel: w318 -> [_ _]
              tunnel: w318 -> [w325 w340]
              tunnel: [w324 w332] -> w317
              frame False {
                n196 = Bundle("x0"=w327, "y0"=w326) -> (w328:cluster{"x0":dbl, "y0":dbl})  [unwired: 1 in]
                n197 = invoke on="Invoke Node" class="XYGraph (strict)" method="Map XY To Coords"(reference=w325, "XY"=w328) -> ("Coords"=w324:T13)  [unwired: 5 in, 6 out]
                n198 = Unbundle(w324) -> ("Horizontal"=w330:i32, "Vertical"=w329:i32)
                n199 = dll-call lib="User32.dll" fn="SetCursorPos"(w330, w329) -> ()  [unwired: 6 in, 2 out]
              }
              frame True {
                n200 = Bundle("x0"=w342, "y0"=w341) -> (w334:cluster{"x0":dbl, "y0":dbl})  [unwired: 1 in]
                n201 = invoke on="Invoke Node" class="XYGraph (strict)" method="Map XY To Coords"(reference=w340, "XY"=w334) -> ("Coords"=w332:T13)  [unwired: 5 in, 6 out]
                n202 = Tick Count (ms)() -> (millisecond timer value=→"initial time":u32)
                n203 = Unbundle(w332) -> ("Horizontal"=w336:i32, "Vertical"=w335:i32)
                n204 = dll-call lib="User32.dll" fn="SetCursorPos"(w336, w335) -> ()  [unwired: 6 in, 2 out]
                n205 = Add(x=1, y=w338) -> (x+y=w337:i32)
              }
            }
          }
        }
        n206 = node-c288() -> ()  [unwired: 1 in, 1 out]
      }
      n207 = Open/Create/Replace File(file path (use dialog)=w98, operation (0:open)=T1."create") -> (refnum out=w100:refnum<file>)  [unwired: 4 in, 2 out]
      n208 = Open/Create/Replace File(file path (use dialog)=w92, operation (0:open)=T1."create") -> (refnum out=w94:refnum<file>)  [unwired: 4 in, 2 out]
      n209 = Open/Create/Replace File(file path (use dialog)=w82, operation (0:open)=T1."create") -> (refnum out=w83:refnum<file>)  [unwired: 4 in, 2 out]
      n210 = Open/Create/Replace File(file path (use dialog)=w79, operation (0:open)=T1."create") -> (refnum out=w80:refnum<file>)  [unwired: 4 in, 2 out]
      n211 = Open/Create/Replace File(file path (use dialog)=w95, operation (0:open)=T1."create") -> (refnum out=w97:refnum<file>)  [unwired: 4 in, 2 out]
      n212 = Close File(refnum=w100) -> ()  [unwired: 1 in, 2 out]
      n213 = Close File(refnum=w94) -> ()  [unwired: 1 in, 2 out]
      n214 = Close File(refnum=w83) -> ()  [unwired: 1 in, 2 out]
      n215 = Close File(refnum=w80) -> ()  [unwired: 1 in, 2 out]
      n216 = Close File(refnum=w97) -> ()  [unwired: 1 in, 2 out]
      n217 = node-c288(w106) -> ()  [unwired: 1 out]
      n218 = call-poly <vilib>:"Close Input Device.vi"("error in (no error)"=w90, "device ID"=w91) -> ()  [unwired: 8 in, 1 out]
      n219 = call "Dispose Kinect.vi"("error in (no error)"=w72, "Queues In"=w69, "References"=w68) -> ("error out"=w73:errorcluster)  [unwired: 2 in]
      n220 = call "IMAQ Dispose"("All Images? (No)"=TRUE, "error in (no error)"=w73) -> ("error out"=w74:errorcluster)  [unwired: 4 in]
      n221 = call <vilib>:"Simple Error Handler.vi"("error in (no error)"=w74) -> ()  [unwired: 4 in, 5 out]
    }
    frame #2 {
      n222 = call "finish.vi"("XYGraph Refnum"=w588) -> ()  [unwired: 11 in]
      n223 = call "Time Delay3"() -> ()  [unwired: 11 in, 1 out]
    }
  }
  n224 = node-c288() -> (w2:T2)  [unwired: 4 in]
  n225 = timed-loop {
    shift-right: [w591] -> _
    shift-left: _ -> [w590]
    timing: w2 -> [_]
    timing-out: [_] -> w1
    stop <- w589 stop-if-true
    n226 = node-c288() -> ()  [unwired: 1 in, 1 out]
    n227 = call "Acquire Sound"() -> ("Data"=w597:dynamicdata)  [unwired: 18 in, 1 out]
    n228 = call "Tone Measurements"("Signals"=w597) -> ("Amplitude"=w596:dynamicdata)  [unwired: 9 in, 1 out]
    n229 = Greater?(x=w596, y=0.105) -> (0:w594:dynamicdata)
    n230 = call "Convert from Dynamic Data"("Dynamic Data Type"=w594) -> ("Scalar"=w591:bool)  [unwired: 3 in]
    n231 = Not(x=w590) -> (.not. x?=w593:bool)
    n232 = And(x=w593, y=w591) -> (x .and. y?=→"click 2":bool)
    n233 = local read "stop"() -> (w589:bool)
    n234 = node-c288() -> ()  [unwired: 1 in, 1 out]
  }
  n235 = node-c288(w1) -> ()  [unwired: 1 out]
  n236 = property class="VI"(reference=w18, error in=w17, "Front Panel Window:Open"=TRUE) -> (reference out=w21:refnum<vi>, error out=w20:errorcluster)
  n237 = Close Reference(reference=w21, error in (no error)=w20) -> ()  [unwired: 1 out]
